vi "Reply.vi"(8 "error in (no error)":errorcluster, 9 "parameter":variant, 10 "request":refnum<class "request.lvclass">, 11 "output in":refnum<class "Output.lvclass">) -> (0 "error out":errorcluster, 3 "output out":refnum<class "Output.lvclass">)   [LabVIEW 2015, in "Output.lvclass"]
uses:
  Output.lvclass
  Request/request.lvclass
  Output.lvclass/Output.ctl
  <vilib>/addons/lv-msgpack/MsgPack Serializer/MsgPackSerializer.lvclass
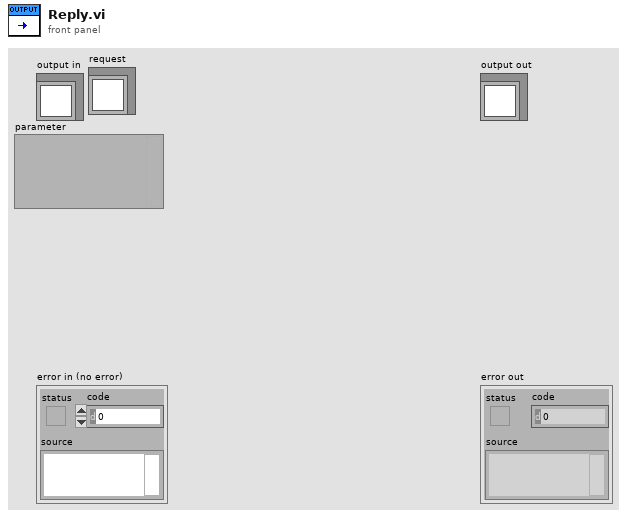
[diagram p1: front panel]
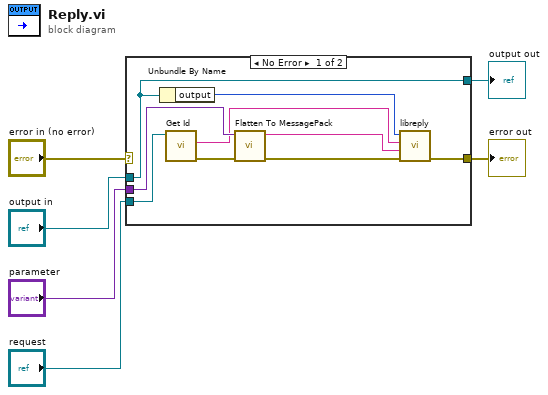
[diagram p0: block diagram]
diagram:
  n1 = case shown="No Error" "error in (no error)" {
    selector: "error in (no error)" -> [_ w17]
    tunnel: [w9 w17] -> w5
    tunnel: [w7 w16] -> w3
    tunnel: "output in" -> [w7 w16]
    tunnel: "parameter" -> [w14 _]
    tunnel: "request" -> [w13 _]
    frame No Error {
      n2 = Unbundle By Name(w7) -> ("output"=w8:i32)
      n3 = call "Get Id.vi"("request in"=w13) -> ("error out"=w15:errorcluster, "id"=w12:string)  [unwired: 8 in, 1 out]
      n4 = call <vilib>:"Flatten To MessagePack.vi"("error in (no error)"=w15, "Data"=w14) -> ("error out"=w10:errorcluster, "MsgPack Data"=w11:string)  [unwired: 8 in]
      n5 = call "libreply.vi"("error in (no error)"=w10, "parameter"=w11, "id"=w12, "output"=w8) -> ("error out"=w9:errorcluster)  [unwired: 7 in]
    }
    frame Error {
    }
  }
  "error out" <- w5
  "output out" <- w3
